vi "Configure DigitalOut.vi"(10 "Samplerate Out":T1=8192 caption="Samplerate" min=10 max=100000000 step=10, 11 "ADALM2000 Handler":u64 caption="Instrument Handle Out") -> (3 "ADALM2000 Handler 2":u64 caption="Instrument Handle Out")   [LabVIEW 2022 SP3]
uses:
  Controls/SampleRateControlDig.ctl
  libm2k_lv.dll
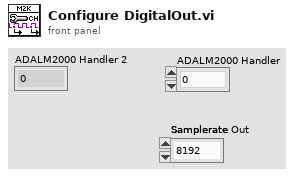
[diagram p1: front panel]
types:
  T1 = typedef "SampleRateControlDig.ctl" = i32
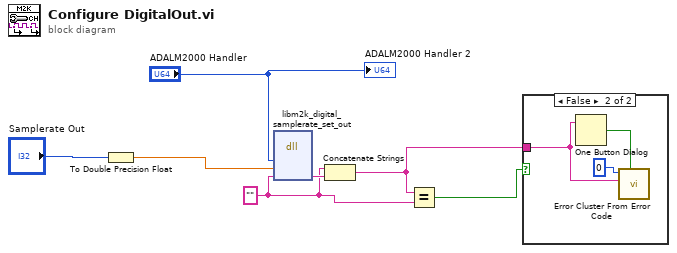
[diagram p0: block diagram]
diagram:
  w5 = ""
  n1 = To Double Precision Float(number="Samplerate Out") -> (double precision float=w7:dbl)
  n2 = dll-call lib="libm2k_lv.*" fn="libm2k_digital_samplerate_set_out"("instance"="ADALM2000 Handler", "samplerate_out"=w7, "err"=w5) -> ("err"=w6:string)  [unwired: 6 in, 2 out]
  n3 = Concatenate Strings(w5, w6) -> (w3:string)
  n4 = Equal?(x=w3, y=w5) -> (x = y?=w4:bool)
  n5 = case shown="False" w4 {
    tunnel: w3 -> [_ w8]
    frame True {
    }
    frame False {
      n6 = One Button Dialog(message=w8) -> (true=w10:bool)  [unwired: 1 in]
      n7 = call <vilib>:"Error Cluster From Error Code.vi"("show call chain? (False)"=w10, "error message (\"\")"=w8, "error code (0)"=0) -> ()  [unwired: 6 in, 1 out]
    }
  }
  "ADALM2000 Handler 2" <- "ADALM2000 Handler"
